vi "Extract All.vi"(8 "Error":errorcluster, 11 "WavBuf":refnum<class "WavBuf.lvclass">) -> (0 "Error Out":errorcluster, 3 "Buffer Out":T1)   [LabVIEW 2020, in "WavBuf.lvclass"]
uses:
  WavBuf.lvclass
  Universal Controls/Waveform_Data.ctl
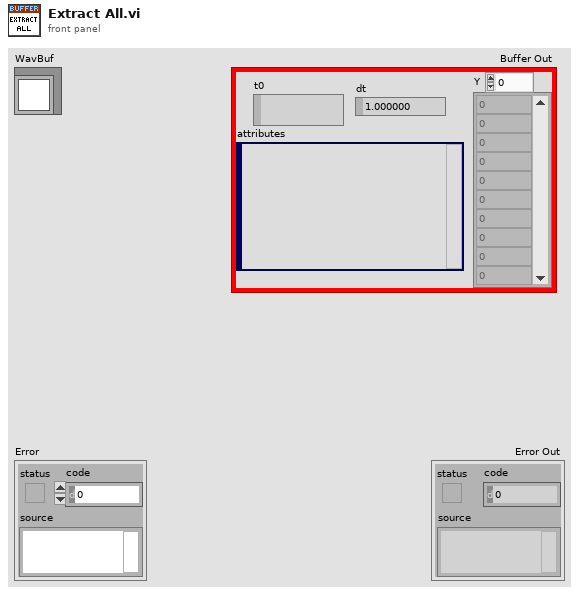
[diagram p1: front panel]
types:
  T1 = typedef "Waveform_Data.ctl" = waveform(dbl)
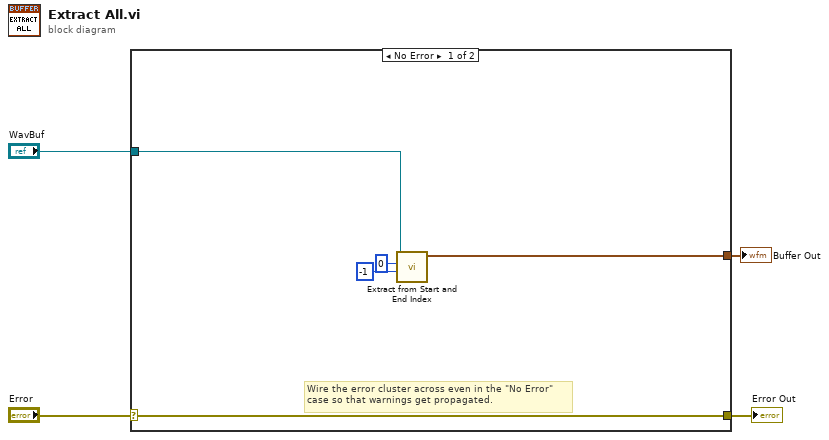
[diagram p0: block diagram]
diagram:
  n1 = case shown="No Error" "Error" {
    selector: "Error" -> [w9 w10]
    tunnel: [w9 w10] -> w3
    tunnel: "WavBuf" -> [w8 _]
    tunnel: [w7 _] -> w1
    frame No Error {
      # "Wire the error cluster across even in the \"No Error\"\ncase so that warnings get propagated."
      n2 = call "Extract from Start and End Index.vi"("End Index\n(-1) Last Point"=-1 ("End Index\n(-1) Last Point"), "Start Index"=0, "WavBuf"=w8) -> ("Buffer Out"=w7:T1)  [unwired: 5 in, 3 out]
    }
    frame Error {
    }
  }
  "Error Out" <- w3
  "Buffer Out" <- w1
